vi "Reset device tester.vi"() -> ()   [LabVIEW 2020]
panel:
  out "Response 2":string
  out "error out":errorcluster
  out "Response":string
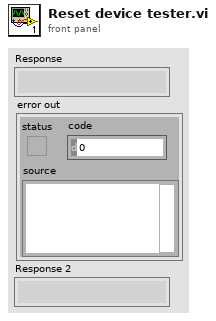
[diagram p1: front panel]
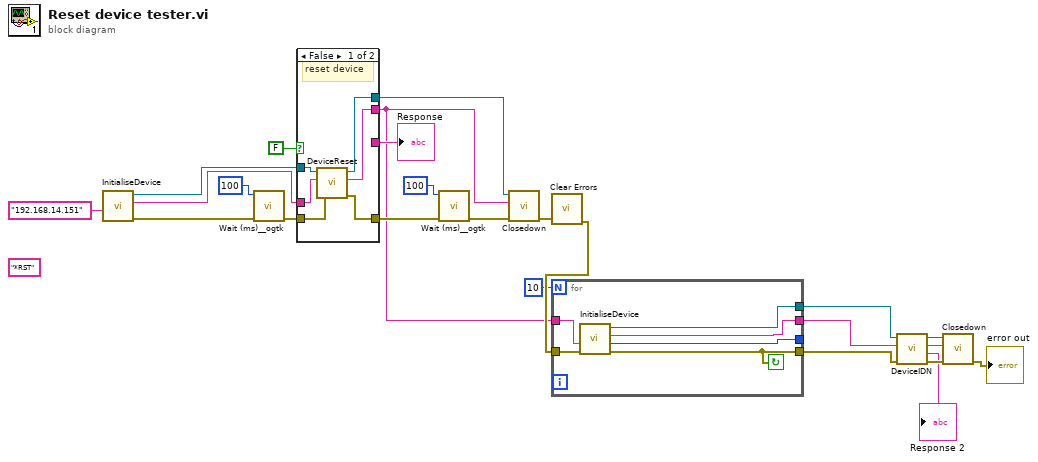
[diagram p0: block diagram]
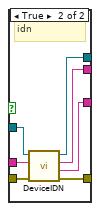
[diagram p2: hidden frame]
diagram:
  (unwired) "*RST" ("Command")
  n1 = call "InitialiseDevice.vi"("PicoMotor IP In"="192.168.14.151") -> ("error out"=w20:errorcluster, "DeviceKey Out"=w18:string, "CmdLib Out"=w19:refnum<k24>)  [unwired: 7 in, 1 out]
  n2 = call <userlib>:"Wait (ms)__ogtk.vi"("error in (no error)"=w20, "milliseconds to wait"=u32 100) -> ("error out"=w17:errorcluster)  [unwired: 8 in, 1 out]
  n3 = case shown="False" FALSE {
    tunnel: w19 -> [w30 w37]
    tunnel: w18 -> [w28 w36]
    tunnel: w17 -> [w27 w35]
    tunnel: [w29 w34] -> w16
    tunnel: [w25 w33] -> w10
    tunnel: [_ w32] -> w15
    tunnel: [w26 w31] -> w14
    frame False {
      # "reset device"
      n4 = call "DeviceReset.vi"("error in (no error)"=w27, "DeviceKey In"=w28, "CmdLib In"=w30) -> ("error out"=w26:errorcluster, "DeviceKey Out"=w25:string, "CmdLib Out"=w29:refnum<k24>)  [unwired: 2 in]
    }
    frame True {
      # "idn"
      n5 = call "DeviceIDN.vi"("error in (no error)"=w35, "DeviceKey In"=w36, "CmdLib In"=w37) -> ("error out"=w31:errorcluster, "Response"=w32:string, "DeviceKey Out"=w33:string, "CmdLib Out"=w34:refnum<k24>)  [unwired: 1 in]
    }
  }
  "Response" <- w15
  n6 = call <userlib>:"Wait (ms)__ogtk.vi"("error in (no error)"=w14, "milliseconds to wait"=u32 100) -> ("error out"=w22:errorcluster)  [unwired: 8 in, 1 out]
  n7 = call "Closedown.vi"("error In"=w22, "DeviceKey In"=w10, "CmdLib In"=w16) -> ("error out"=w12:errorcluster)  [unwired: 8 in]
  n8 = call <vilib>:"Clear Errors.vi"("error in (no error)"=w12) -> ("error out"=w11:errorcluster)  [unwired: 5 in, 1 out]
  n9 = for {
    N: 10 -> [_]
    tunnel: [w42] -> w8
    tunnel: [w40] -> _
    tunnel: w11 -> [w39]
    tunnel: [w38] -> w6
    tunnel: w10 -> [w43]
    tunnel: [w41] -> w7
    stop <- w38 continue-if-true
    n10 = call "InitialiseDevice.vi"("error In"=w39, "PicoMotor IP In"=w43) -> ("error out"=w38:errorcluster, "Device Address Out"=w40:i32, "DeviceKey Out"=w41:string, "CmdLib Out"=w42:refnum<k24>)  [unwired: 6 in]
  }
  n11 = call "DeviceIDN.vi"("error in (no error)"=w6, "DeviceKey In"=w7, "CmdLib In"=w8) -> ("error out"=w3:errorcluster, "Response"=→"Response 2":string, "DeviceKey Out"=w4:string, "CmdLib Out"=w5:refnum<k24>)  [unwired: 1 in]
  n12 = call "Closedown.vi"("error In"=w3, "DeviceKey In"=w4, "CmdLib In"=w5) -> ("error out"=→"error out":errorcluster)  [unwired: 8 in]
